vi "MOVE(SubVI).vi"(8 "Move Direction":i32[](array[numeric]), 9 "former position":i32[](array[numeric]), 10 "boarder":i32[][](array[numeric]), 11 "key in":T1(ring)) -> (2 "Move Direction out":i32[](array[numeric]), 3 "position":i32[](array[numeric]))   [LabVIEW 2014]
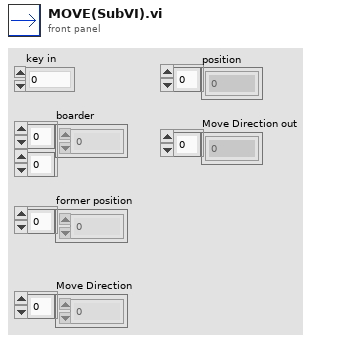
[diagram p1: front panel]
types:
  T1 = enum16{"0", "1", "2", "3", "4", "5", "6", "7", "8", "9", "A", "B", "C", "D", "E", "F", "G", "H", "I", "J", "K", "L", "M", "N", "O", "P", "Q", "R", "S", "T", "U", "V", "W", "X", "Y", "Z", "F1", "F2", "F3", "F4", "F5", "F6", "F7", "F8", "F9", "F10", "F11", "F12", "F13", "F14", "F15", "ADD", "BACK", "BACKSLASH", "CAPITAL", "COMMA", "DECIMAL", "DELETE", "DIVIDE", "DOWN", "END", "EQUALS", "ESCAPE", "GRAVE (`)", "HOME", "INSERT", "LBRACKET", "LCONTROL", "LEFT", "L ALT", "LSHIFT", "LWIN", "MINUS", "MULTIPLY", "NEXT", "NUMLOCK", "NUMPAD_0", "NUMPAD_1", "NUMPAD_2", "NUMPAD_3", "NUMPAD_4", "NUMPAD_5", "NUMPAD_6", "NUMPAD_7", "NUMPAD_8", "NUMPAD_9", "PAUSE", "PERIOD", "PRIOR (PG UP)", "RBRACKET", "RCONTROL", "RETURN", "RIGHT", "R ALT", "RSHIFT", "RWIN", "SCROLL", "SEMICOLON", "SLASH", "SPACE", "SUBTRACT", "TAB", "UP", "ENTER (num pad)", "' (quote)"}
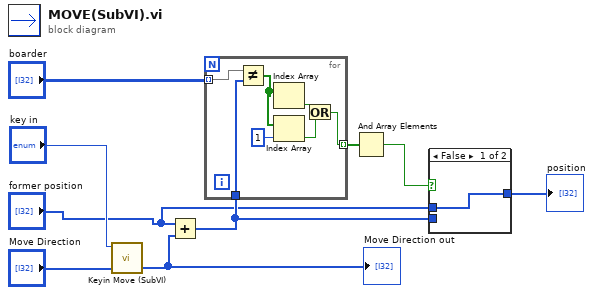
[diagram p0: block diagram]
diagram:
  n1 = call "Keyin Move (SubVI).vi"("Move Direction"="Move Direction", "keyType 3"="key in") -> ("Move Direction out"=w6:i32[])  [unwired: 9 in]
  "Move Direction out" <- w6
  n2 = Add(x="former position", y=w6) -> (x+y=w2:i32[])
  n3 = for {
    tunnel: "boarder" -> [w16] mode=indexing
    tunnel: w2 -> [w15]
    tunnel: [w10] -> w9 mode=indexing
    n4 = Not Equal?(x=w16, y=w15) -> (x != y?=w14:bool[])
    n5 = Index Array(array=w14) -> (element=w11:bool)  [unwired: 1 in]
    n6 = Index Array(array=w14, index=1) -> (element=w12:bool)
    n7 = Or(x=w11, y=w12) -> (x .or. y?=w10:bool)
  }
  n8 = And Array Elements(Boolean array=w9) -> (logical AND=w7:bool)
  n9 = case shown="False" w7 {
    tunnel: [w17 w18] -> w3
    tunnel: w2 -> [_ w18]
    tunnel: "former position" -> [w17 _]
    frame False {
    }
    frame True {
    }
  }
  "position" <- w3
